vi "Sub Super Duper_7_24_12a_PD.vi"(0 "VISA resource name":refnum<visa-resource-name>="GPIB0::17::INSTR", 1 "Sample Properties:":T5 {"Date Created" format="%<%Y/%m/%d>T"}, 2 "TRF Cluster":T6={"Step 4"=-38.0, "# of Loops"=1.0, "Transfer 2"=FALSE, "Start 4"=-2.0, "Total Points 2"=2, "Start 3"=40.0, "Stop 2"=-40.0, "Step 3"=-1.0, "Loop Step"=0.0, "Integration Time 3"=0, "Loop Wait"=0.0, "First Step"=0.0} {"Loop Wait" format="%<%H:%M:%S>t"; "Integration Time 3" scale=0.0..2.0; "Step 3" format="%.2f"; "Stop 2" format="%.2f"; "Start 3" format="%.2f"; "Start 4" format="%.2f"; "Step 4" format="%.2f"}, 3 "TSP Cluster":T7={"Transport"=FALSE, "Start 2"=0.0, "Stop 3"=-60.0, "Step 2"=-1.0, "Start"=0.0, "Step"=-10.0, "Total Points"=7, "Integration Time"=0} {"Integration Time" scale=0.0..2.0; "Step" format="%.2f"; "Start" format="%.2f"; "Step 2" format="%.2f"; "Stop 3" format="%.2f"; "Start 2" format="%.2f"}, 4 "Compliance Cluster":T2={"Var1 sweep settings"={"sweep spacing (linear: 0)"=0, "sweep mode"=FALSE, "compliance (V)"=100.0, "compliance (A)"=0.001}, "Var1 sweep settings 2"={"sweep spacing (linear: 0)"=0, "sweep mode"=FALSE, "compliance (V)"=100.0, "compliance (A)"=0.001}, "Var2 step settings 2"={"compliance (A)"=0.001, "compliance (V)"=100.0}, "Var2 step settings"={"compliance (A)"=0.001, "compliance (V)"=100.0}} {"Var2 step settings"."compliance (V)" format="%.2f"; "Var2 step settings"."compliance (A)" format="%^.2e"; "Var2 step settings 2"."compliance (V)" format="%.2f"; "Var2 step settings 2"."compliance (A)" format="%^.2e"; "Var1 sweep settings 2"."compliance (A)" format="%^.2e"; "Var1 sweep settings 2"."compliance (V)" format="%.2f"; "Var1 sweep settings 2"."sweep spacing (linear: 0)" items=["linear", "log 10", "log 25", "log 50"]; "Var1 sweep settings"."compliance (A)" format="%^.2e"; "Var1 sweep settings"."compliance (V)" format="%.2f"; "Var1 sweep settings"."sweep spacing (linear: 0)" items=["linear", "log 10", "log 25", "log 50"]}, 5 "error in":errorcluster, 6 "Saved Folder:":path=path "C:/1DATA/2011", 7 "Wait Cluster":T1 {"Wait Time (s)" format="%.1g"; "Wait Countdown" format="%<%H:%M:%S%1u>t"}, 9 "Stop \nCountdown":bool, 11 "Loop Count":dbl) -> (8 "Status Indicator":bool, 14 "VISA resource name out":refnum<visa-resource-name>, 15 "TRF Path":path, 16 "TSP Path":path, 17 "Graph Cluster":T3, 18 "Char Cluster":T4, 19 "error out":errorcluster)   [LabVIEW 2011]
uses:
  <vilib>/Platform/TimedLoop/XDataNode/wakeup.ctl
  <vilib>/Platform/TimedLoop/XDataNode/XDNodeRunTimeDep.lvlib
  <vilib>/Platform/TimedLoop/XDataNode/nitl_modes.ctl
  <vilib>/Platform/TimedLoop/XDataNode/timing_clust.ctl
  <vilib>/Platform/TimedLoop/XDataNode/XDataNode.xnode
panel:
  in  "Transport Temp":cluster{"trace":dbl[], "trace":dbl[]}(graph)
  in  "Graph":cluster{dbl[], "trace":dbl[]}[](graph) caption="Transfer"
  # "Vg Sweep"
  # "Vd Step"
  # "Loops and Integration Time"
  # "Device Characteristics"
  # "Sample Properties:"
  # "%"
  # "nm"
  # "Device Properties:"
  # "um"
  # "um"
  # "Vg Step"
  # "Vd Step"
  # "Integration Time"
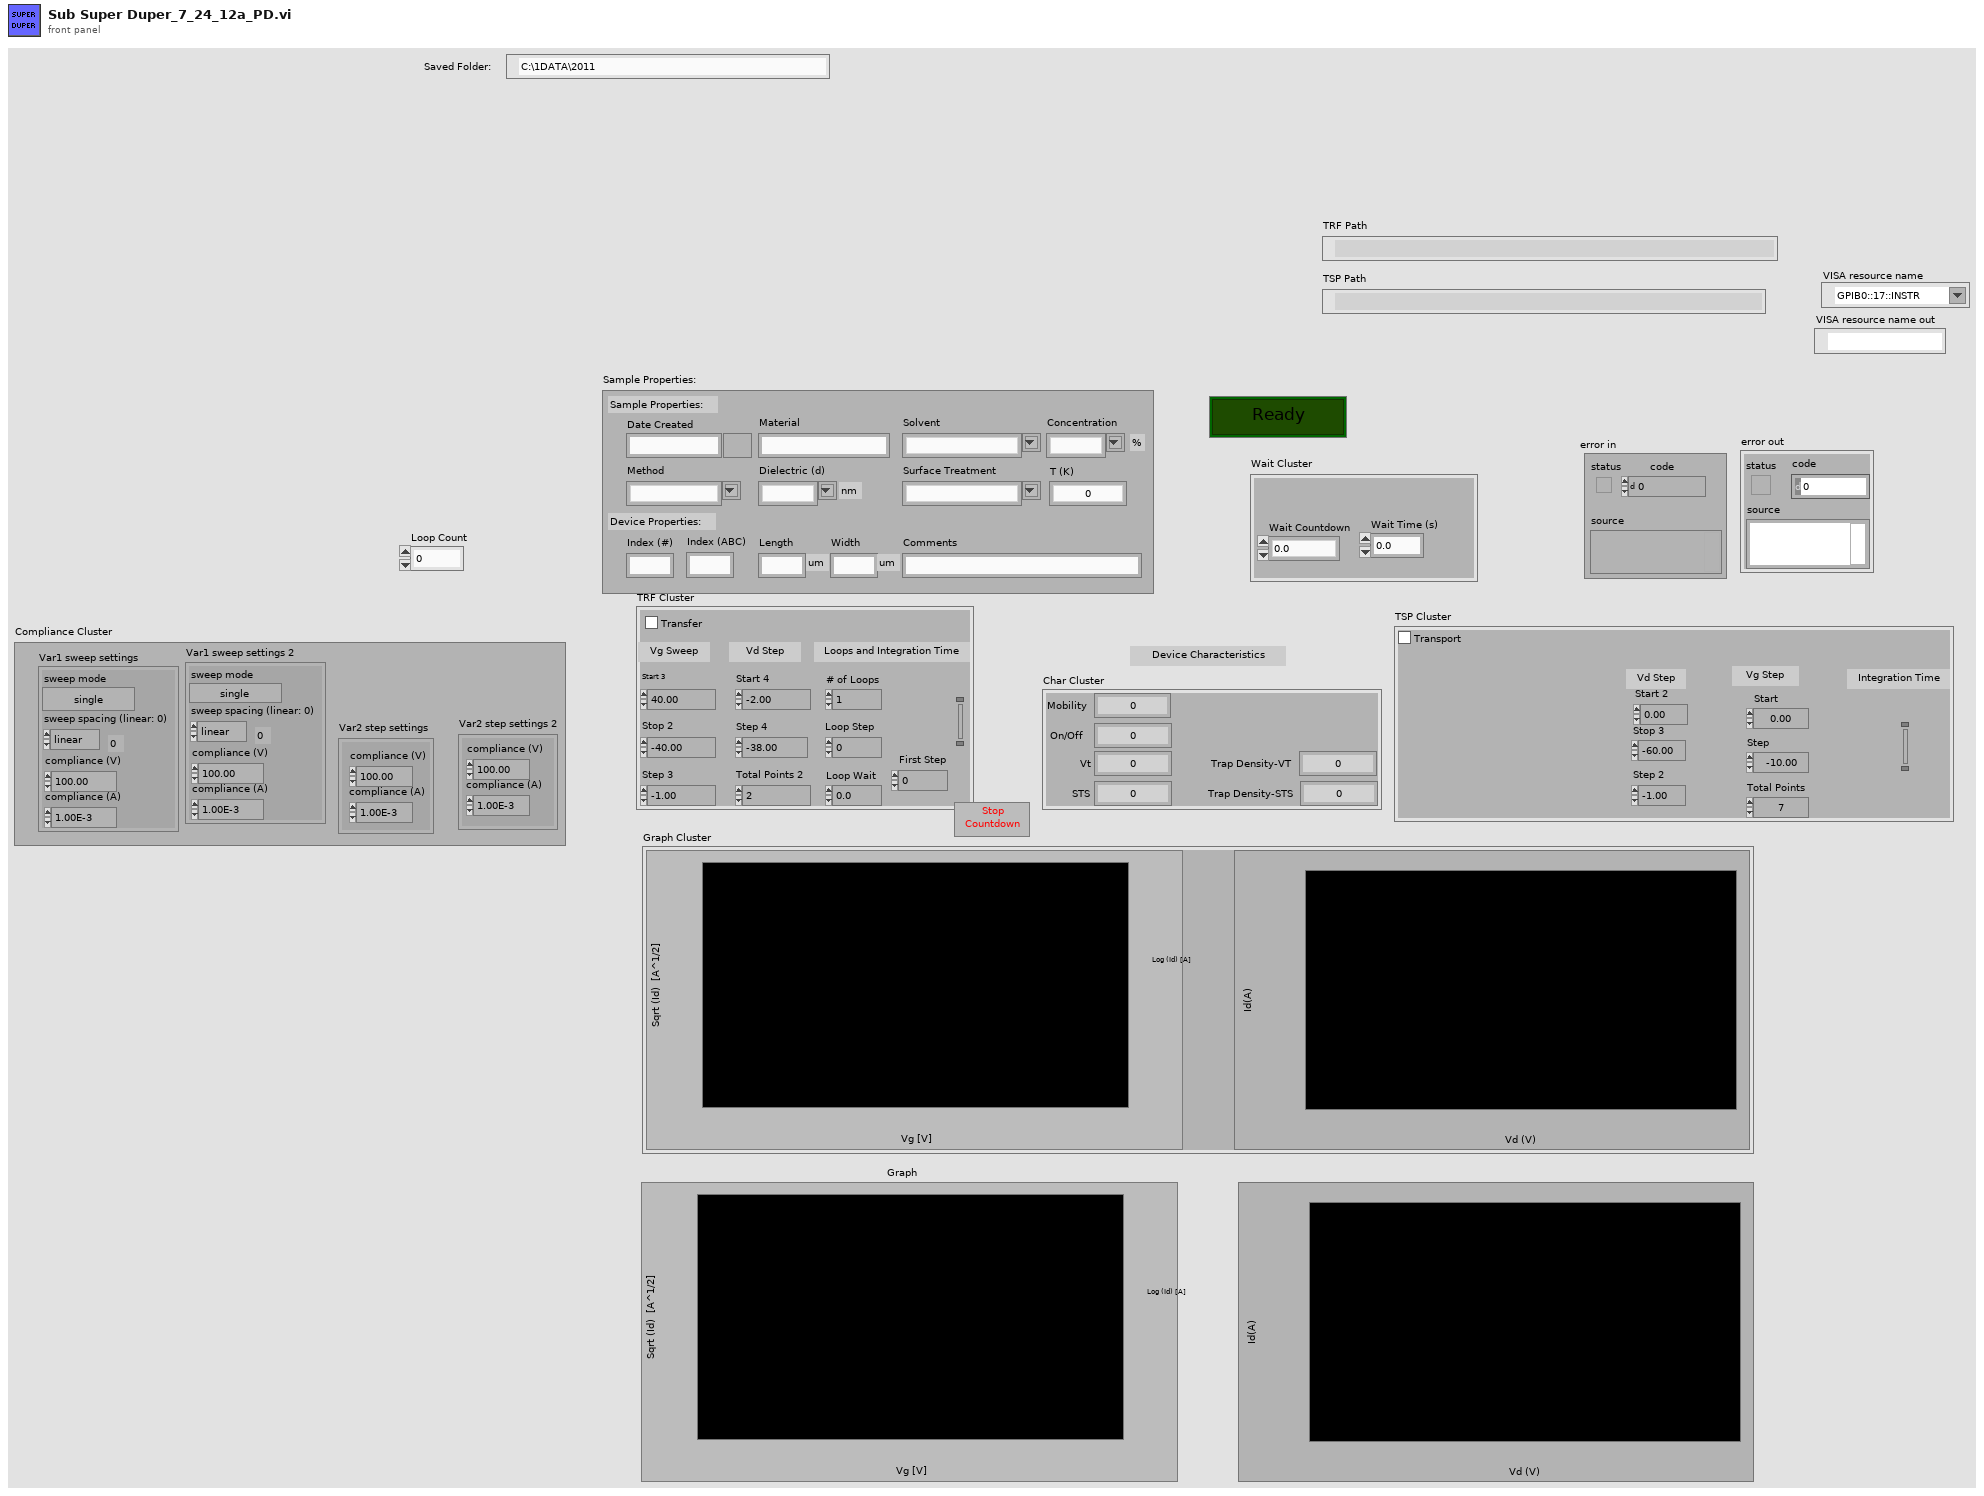
[diagram p1: front panel]
types:
  T1 = cluster{"Wait Countdown":dbl, "Wait Time (s)":dbl}
  T2 = cluster{"Var1 sweep settings":cluster{"sweep spacing (linear: 0)":u16, "sweep mode":bool, "compliance (V)":dbl, "compliance (A)":dbl}, "Var1 sweep settings 2":cluster{"sweep spacing (linear: 0)":u16, "sweep mode":bool, "compliance (V)":dbl, "compliance (A)":dbl}, "Var2 step settings 2":cluster{"compliance (A)":dbl, "compliance (V)":dbl}, "Var2 step settings":cluster{"compliance (A)":dbl, "compliance (V)":dbl}}
  T3 = cluster{"Transfer":cluster{dbl[], "trace":dbl[]}[], "Transport":cluster{"trace":dbl[], "trace":dbl[]}}
  T4 = cluster{"Mobility":dbl, "On/Off ":dbl, "Vt":dbl, "STS":dbl, "Trap Density-STS":dbl, "Trap Density-VT":dbl}
  T5 = cluster{"Date Created":timestamp, "Material":string, "Solvent":string, "Concentration":string, "Method":string, "Dielectric (d)":string, "Index (#)":string, "Index (ABC)":string, "Length":string, "Width":string, "Surface Treatment":string, "Comments":string, "T (K)":dbl}
  T6 = cluster{"Step 4":dbl, "# of Loops":dbl, "Transfer 2":bool, "Start 4":dbl, "Total Points 2":u16, "Start 3":dbl, "Stop 2":dbl, "Step 3":dbl, "Loop Step":dbl, "Integration Time 3":u32, "Loop Wait":dbl, "First Step":dbl}
  T7 = cluster{"Transport":bool, "Start 2":dbl, "Stop 3":dbl, "Step 2":dbl, "Start":dbl, "Step":dbl, "Total Points":u16, "Integration Time":u32}
  T8 = typedef "XDNodeRunTimeDep.lvlib/timing_clust.ctl" = cluster{"Expected End [f-1]":u64, "Actual End [f-1]":u64, "Finished Late? [f-1]":bool, "Expected End [i-1]":u64, "Actual End [i-1]":u64, "Finished Late? [i-1]":bool, "Expected Start [i]":u64, "Actual Start [i]":u64, "Expected Start [f]":u64, "Actual Start [f]":u64, "Source Name":string, "Structure Name":string, "Period":i64, "Deadline":i64, "Offset":i64, "Start":i64, "Priority":i32, "Timeout":i32, "Mode":T9, "Wakeup Reason":T10, "Error":errorcluster, "Source Type":string, "Secondary Source Type":string, "Global End Time":u64, "Global Start Time":u64, "Frame Duration":u64, "Iteration Duration":u64, "Assigned CPU":i32, "I/O Scan Engine Mode":u32}
  T9 = typedef "XDNodeRunTimeDep.lvlib/nitl_modes.ctl" = enum32{"No Change", "Process missed periods, maintain original phase", "Discard missed periods, maintain original phase", "Process missed periods, ignore original phase", "Discard missed periods, ignore original phase"}
  T10 = typedef "XDNodeRunTimeDep.lvlib/wakeup.ctl" = enum32{"Normal", "Aborted", "Asynchronous wakeup", "Timing source error", "Timed loop error", "Timeout"}
  T11 = cluster{"sweep spacing (linear: 0)":u16, "sweep mode":bool, "compliance (V)":dbl, "compliance (A)":dbl}
  T12 = cluster{"compliance (A)":dbl, "compliance (V)":dbl}
  T13 = cluster{"Start 3":dbl, "Stop 2":dbl, "Step 3":dbl, "sweep spacing (linear: 0)":u16, "sweep mode":bool, "compliance (V)":dbl, "compliance (A)":dbl}
  T14 = cluster{"compliance (A)":dbl, "compliance (V)":dbl, "Start 4":dbl, "Total Points 2":u16, dbl}
  T15 = cluster{"Mobility":dbl, "On/Off Current":dbl, "Vt":dbl, "STS":dbl, "Trap Density-VT":dbl, "Trap Density-STS":dbl}
  T16 = cluster{"Start 2":dbl, "Stop 3":dbl, "Step 2":dbl, "sweep spacing (linear: 0)":u16, "sweep mode":bool, "compliance (V)":dbl, "compliance (A)":dbl}
  T17 = cluster{"compliance (A)":dbl, "compliance (V)":dbl, "Start":dbl, "Total Points":u16, "Step":dbl}
  T18 = cluster{"Graph":cluster{dbl[], "trace":dbl[]}[], "Transport Temp":cluster{"trace":dbl[], "trace":dbl[]}}
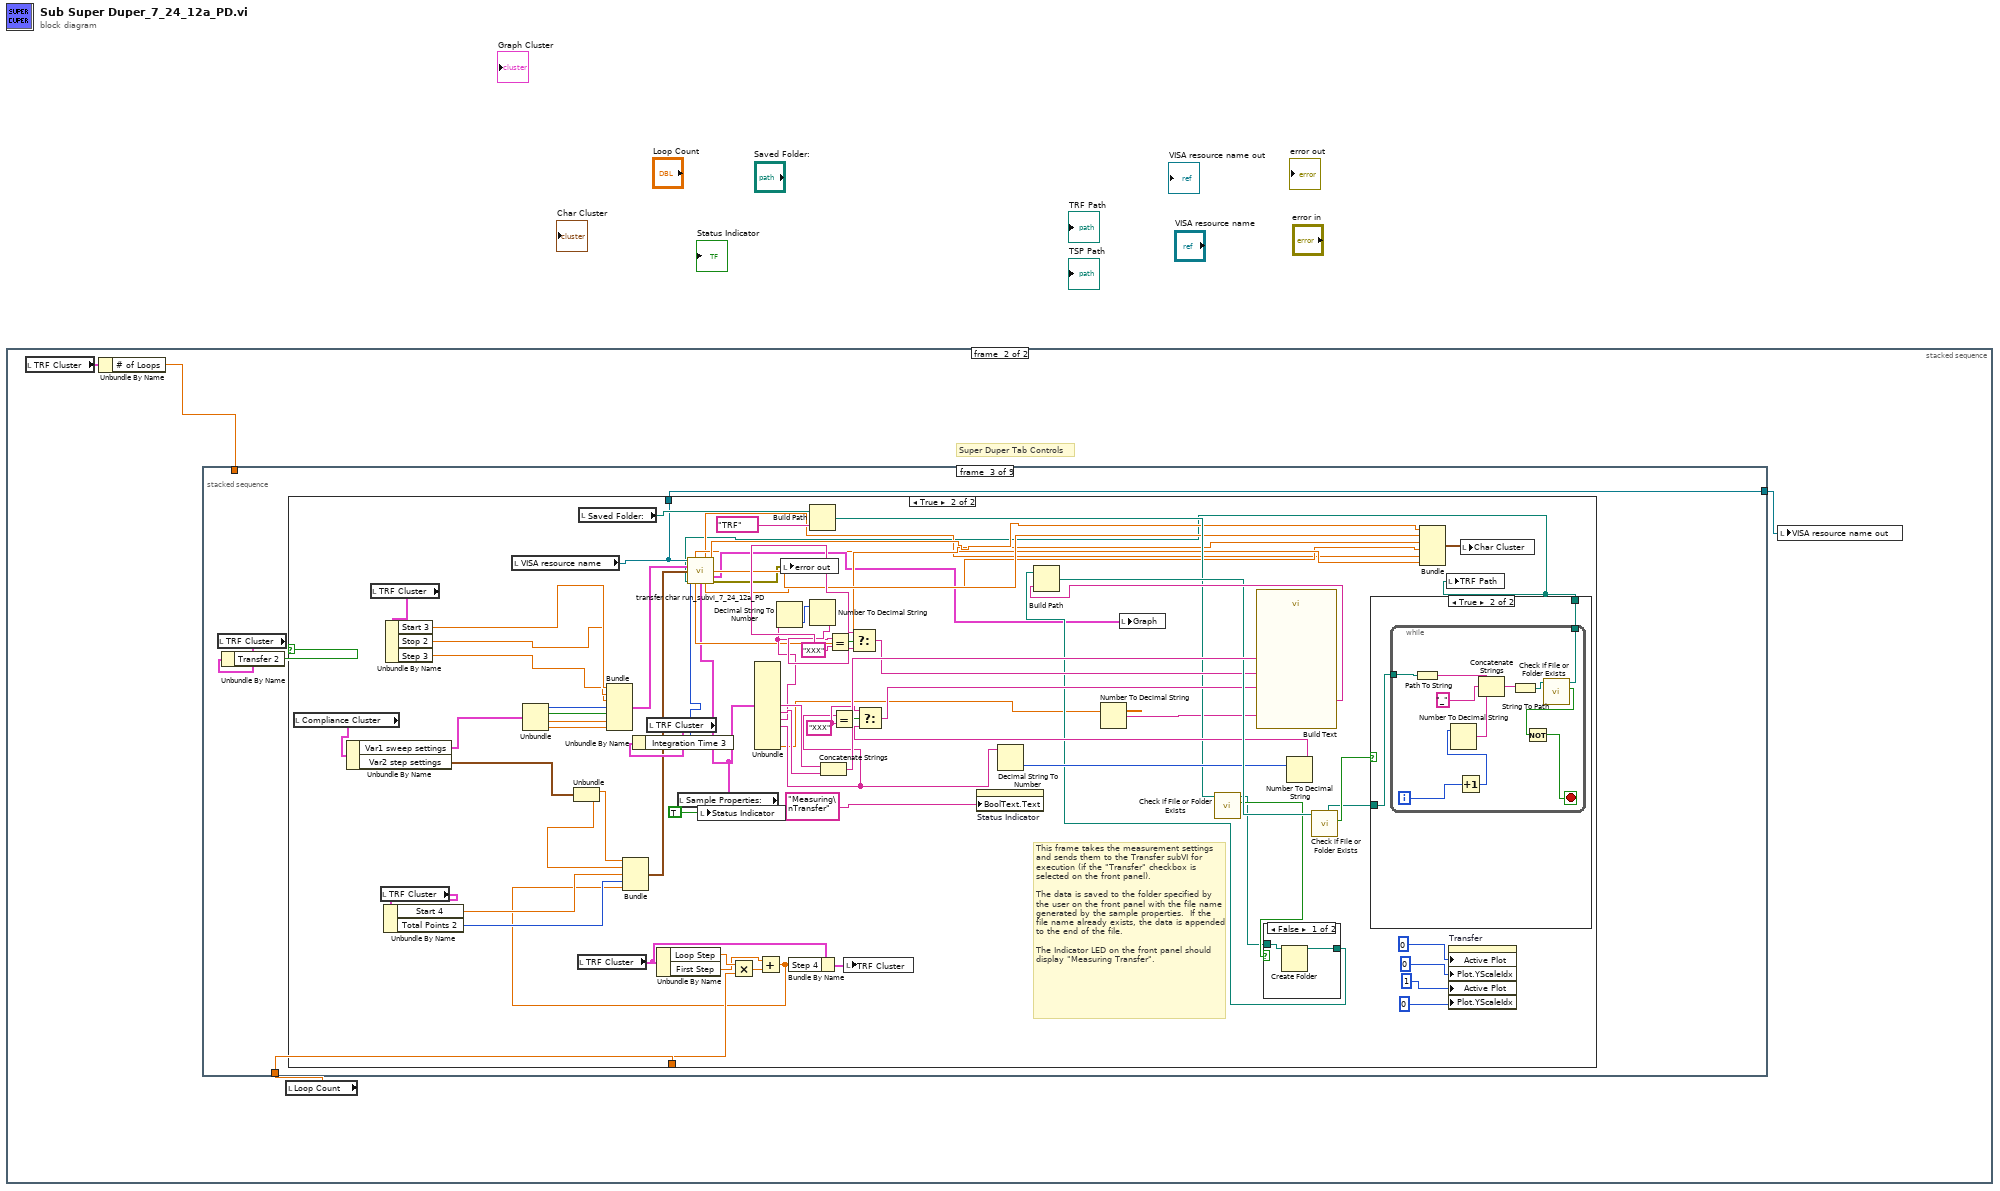
[diagram p0: block diagram]
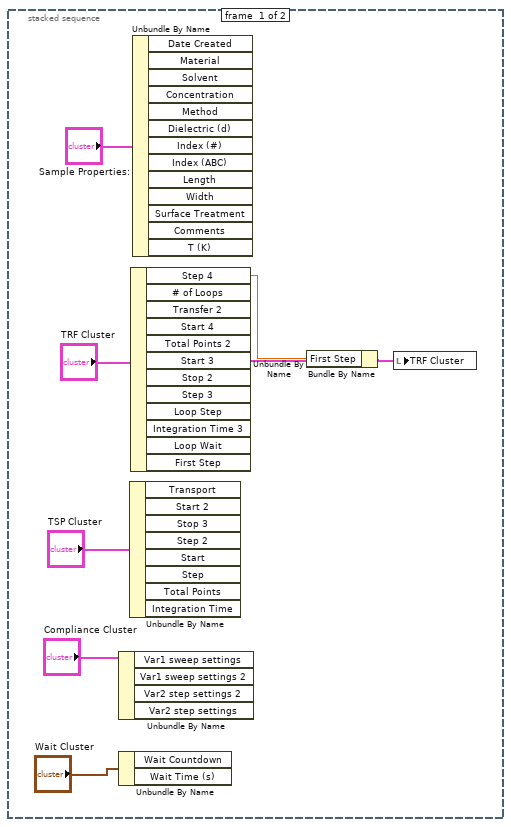
[diagram p2: hidden frame]
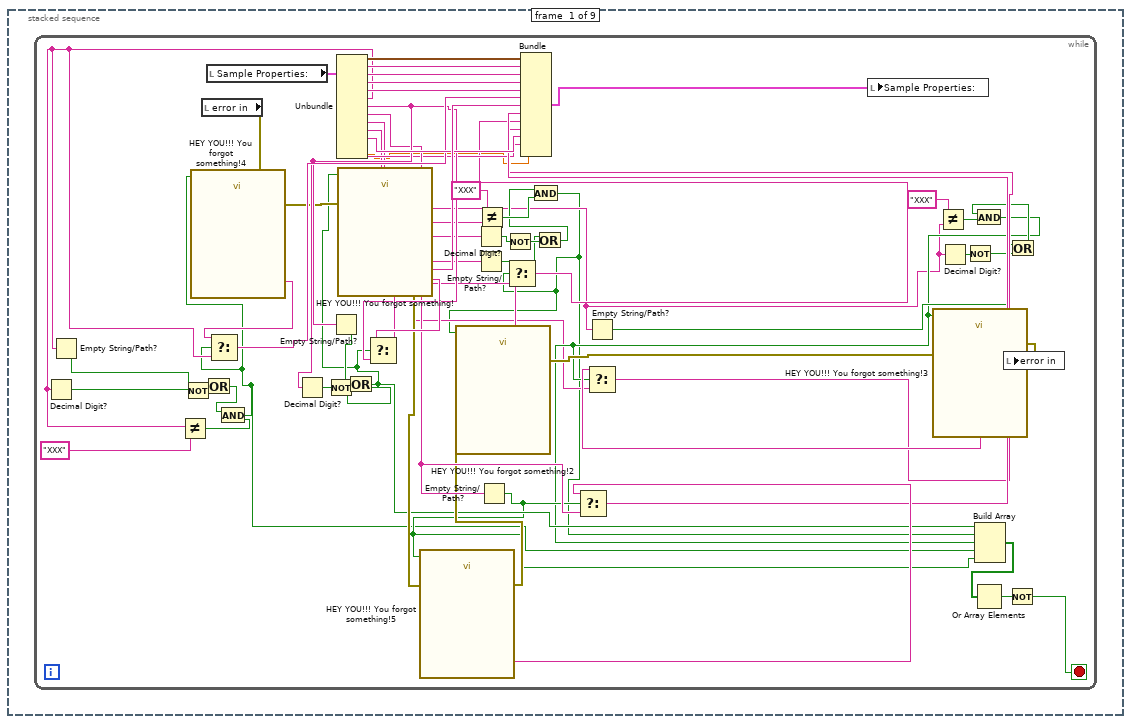
[diagram p3: hidden frame]
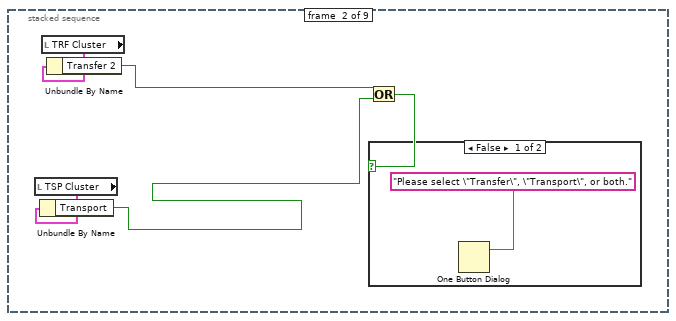
[diagram p4: hidden frame]
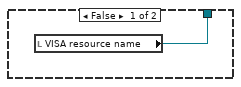
[diagram p6: hidden frame]
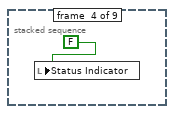
[diagram p9: hidden frame]
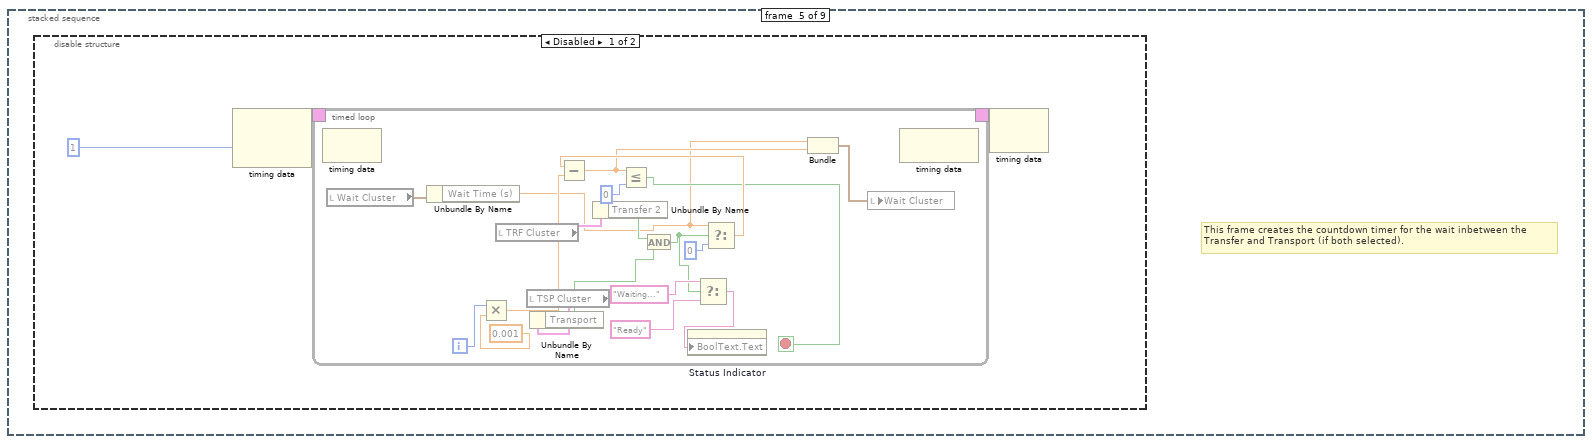
[diagram p10: hidden frame]
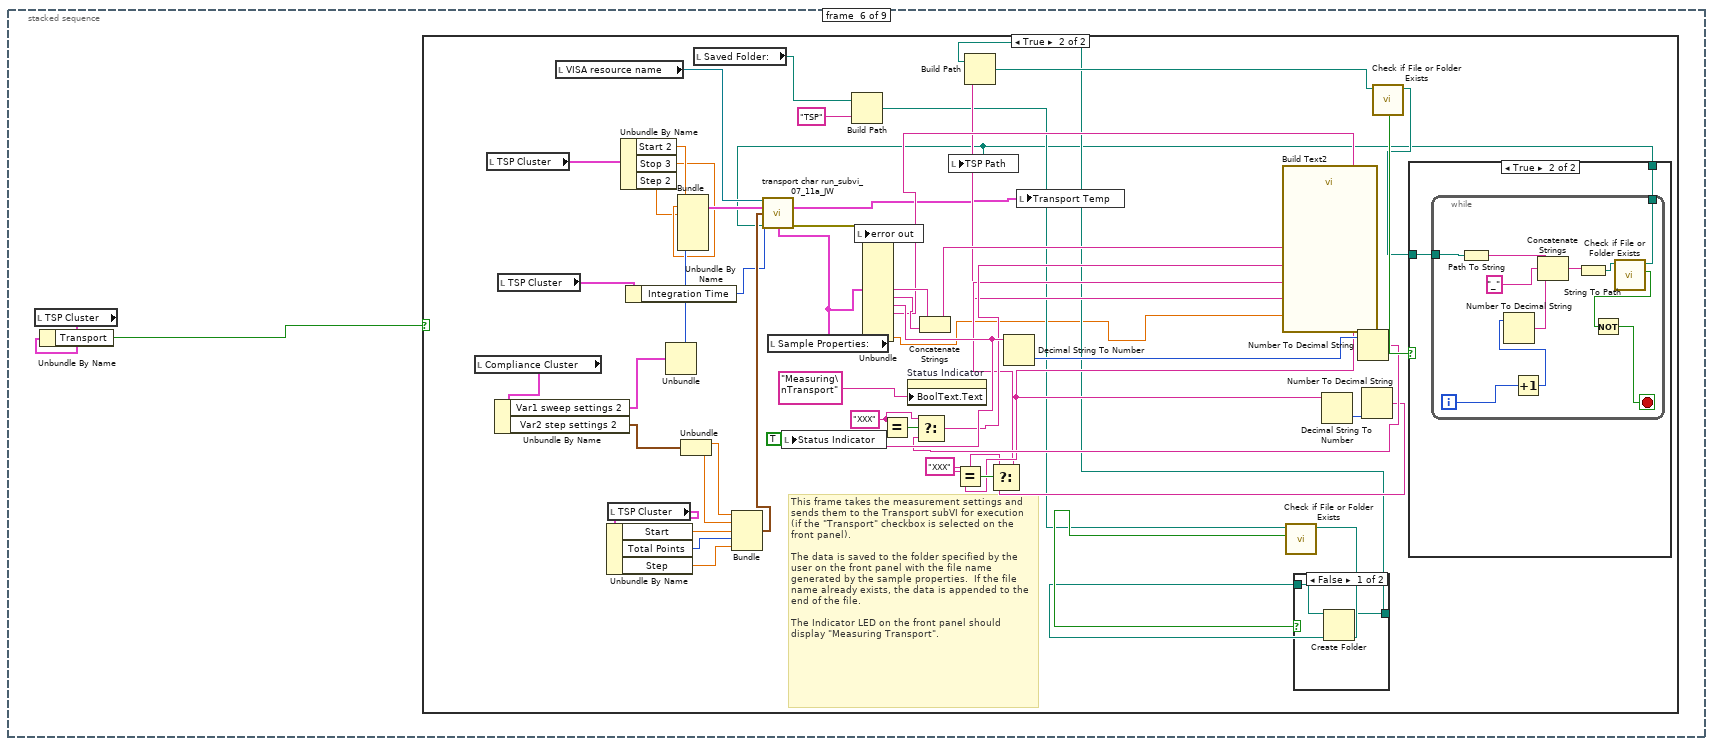
[diagram p12: hidden frame]
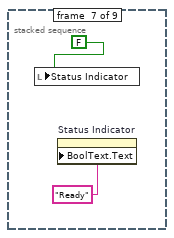
[diagram p16: hidden frame]
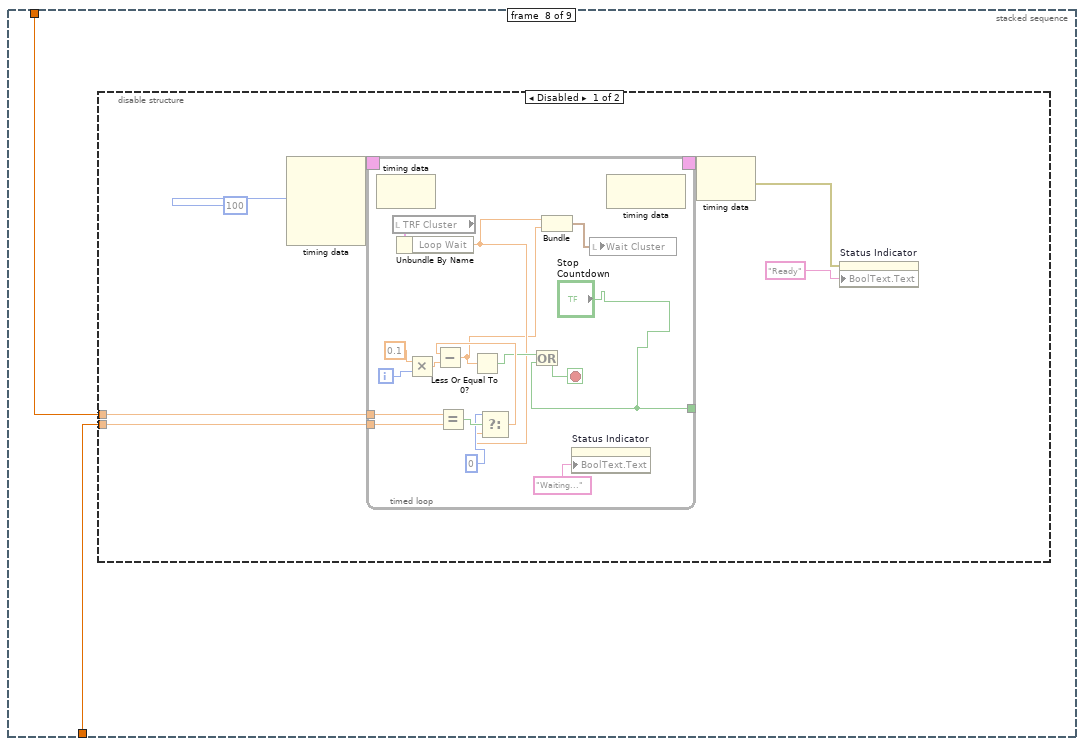
[diagram p17: hidden frame]
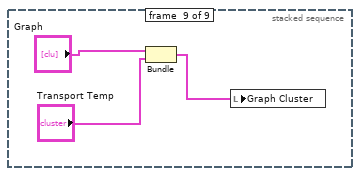
[diagram p19: hidden frame]
diagram:
  n1 = stacked-sequence {
    frame #0 {
      n2 = Unbundle By Name("Compliance Cluster") -> ()  [unwired: 4 out]
      n3 = Unbundle By Name("Wait Cluster") -> ()  [unwired: 2 out]
      n4 = Unbundle By Name("TSP Cluster") -> ()  [unwired: 8 out]
      n5 = Unbundle By Name("TRF Cluster") -> ("Step 4"=w7:dbl)  [unwired: 11 out]
      n6 = Unbundle By Name("Sample Properties:") -> ()  [unwired: 13 out]
      n7 = Bundle By Name(cluster="TRF Cluster", "First Step"=w7) -> (w5:T6)
      n8 = local write "TRF Cluster"(w5) -> ()
    }
    frame #1 {
      # "Super Duper Tab Controls"
      n9 = local read "TRF Cluster"() -> (w11:T6)
      n10 = Unbundle By Name(w11) -> ("# of Loops"=w10:dbl)
      n11 = local read "Loop Count"() -> (w8:dbl)
      n12 = stacked-sequence {
        tunnel: w8 -> [_ _ w81 _ _ _ _ w277 _]
        tunnel: w10 -> [_ _ _ _ _ _ _ w276 _]
        tunnel: [_ _ w78 _ _ _ _ _ _] -> w9
        frame #0 {
          n13 = while {
            stop <- w37 stop-if-true
            n14 = local read "error in"() -> (w43:errorcluster)
            n15 = local read "Sample Properties:"() -> (w66:T5)
            n16 = Unbundle(w66) -> ("Date Created"=w67:timestamp, "Material"=w68:string, "Solvent"=w69:string, "Concentration"=w70:string, "Method"=w71:string, "Dielectric (d)"=w26:string, "Index (#)"=w56:string, "Index (ABC)"=w53:string, "Length"=w21:string, "Width"=w14:string, "Surface Treatment"=w59:string, "Comments"=w51:string, "T (K)"=w12:dbl)
            n17 = Decimal Digit?(1:w26) -> (0:w34:bool)
            n18 = Empty String/Path?(string/path=w26) -> (empty?=w28:bool)
            n19 = Not Equal?(x=w26, y="XXX") -> (x != y?=w25:bool)
            n20 = Not(x=w34) -> (.not. x?=w31:bool)
            n21 = Or(x=w28, y=w31) -> (x .or. y?=w24:bool)
            n22 = And(x=w24, y=w25) -> (x .and. y?=w23:bool)
            n23 = call "HEY YOU!!! You forgot something!4"("Enable"=w23, "error in (no error)"=w43) -> ("Dielectric (d)"=w58:string, "error out"=w42:errorcluster)  [unwired: 15 in, 1 out]
            n24 = Select(t=w58, s=w23, f=w26) -> (s? t:f=w57:string)
            n25 = Decimal Digit?(1:w56) -> (0:w47:bool)
            n26 = Not(x=w47) -> (.not. x?=w46:bool)
            n27 = Empty String/Path?(string/path=w56) -> (empty?=w55:bool)
            n28 = Or(x=w55, y=w46) -> (x .or. y?=w41:bool)
            n29 = call "HEY YOU!!! You forgot something!"("Enable"=w41, "error in (no error)"=w42) -> ("Index (#)"=w65:string, "error out"=w45:errorcluster)  [unwired: 15 in, 1 out]
            n30 = Select(t=w65, s=w41, f=w56) -> (s? t:f=w62:string)
            n31 = Decimal Digit?(1:w21) -> (0:w36:bool)
            n32 = Empty String/Path?(string/path=w21) -> (empty?=w30:bool)
            n33 = Not Equal?(x="XXX", y=w21) -> (x != y?=w20:bool)
            n34 = Empty String/Path?(string/path=w53) -> (empty?=w40:bool)
            n35 = call "HEY YOU!!! You forgot something!5"("Enable"=w40, "error in (no error)"=w45) -> ("Index (ABC)"=w54:string, "error out"=w44:errorcluster)  [unwired: 15 in, 1 out]
            n36 = Not(x=w36) -> (.not. x?=w33:bool)
            n37 = Or(x=w30, y=w33) -> (x .or. y?=w19:bool)
            n38 = And(x=w19, y=w20) -> (x .and. y?=w13:bool)
            n39 = call "HEY YOU!!! You forgot something!2"("Enable"=w13, "error in (no error)"=w44) -> ("Length"=w64:string, "error out"=w61:errorcluster)  [unwired: 15 in, 1 out]
            n40 = Select(t=w64, s=w13, f=w21) -> (s? t:f=w50:string)
            n41 = Select(t=w54, s=w40, f=w53) -> (s? t:f=w52:string)
            n42 = Empty String/Path?(string/path=w14) -> (empty?=w29:bool)
            n43 = Not Equal?(x="XXX", y=w14) -> (x != y?=w18:bool)
            n44 = Decimal Digit?(1:w14) -> (0:w35:bool)
            n45 = Not(x=w35) -> (.not. x?=w32:bool)
            n46 = Or(x=w29, y=w32) -> (x .or. y?=w17:bool)
            n47 = And(x=w17, y=w18) -> (x .and. y?=w16:bool)
            n48 = call "HEY YOU!!! You forgot something!3"("Enable"=w16, "error in (no error)"=w61) -> ("Width"=w63:string, "error out"=w60:errorcluster)  [unwired: 15 in, 1 out]
            n49 = Select(t=w63, s=w16, f=w14) -> (s? t:f=w49:string)
            n50 = Bundle("Date Created"=w67, "Material"=w68, "Solvent"=w69, "Concentration"=w70, "Method"=w71, "Dielectric (d)"=w57, "Index (#)"=w62, "Index (ABC)"=w52, "Length"=w50, "Width"=w49, "Surface Treatment"=w59, "Comments"=w51, "T (K)"=w12) -> (w48:T5)  [unwired: 1 in]
            n51 = local write "Sample Properties:"(w48) -> ()
            n52 = Build Array(w41, w13, w16, w23, w40) -> (w39:bool[])
            n53 = Or Array Elements(Boolean array=w39) -> (logical OR=w38:bool)
            n54 = local write "error in"(w60) -> ()
            n55 = Not(x=w38) -> (.not. x?=w37:bool)
          }
        }
        frame #1 {
          n56 = local read "TSP Cluster"() -> (w73:T7)
          n57 = Unbundle By Name(w73) -> ("Transport"=w72:bool)
          n58 = local read "TRF Cluster"() -> (w75:T6)
          n59 = Unbundle By Name(w75) -> ("Transfer 2"=w74:bool)
          n60 = Or(x=w74, y=w72) -> (x .or. y?=w76:bool)
          n61 = case shown="False" w76 {
            frame False {
              n62 = One Button Dialog(message="Please select \"Transfer\", \"Transport\", or both.") -> ()  [unwired: 1 in, 1 out]
            }
            frame True {
            }
          }
        }
        frame #2 {
          n63 = local read "TRF Cluster"() -> (w79:T6)
          n64 = Unbundle By Name(w79) -> ("Transfer 2"=w80:bool)
          n65 = case shown="True" w80 {
            tunnel: w81 -> [_ w98]
            tunnel: [w82 w89] -> w78
            frame False {
              n66 = local read "VISA resource name"() -> (w82:refnum<visa-resource-name>)
            }
            frame True {
              w132 = "XXX"
              w136 = "XXX"
              # "This frame takes the measurement settings and sends them to the Transfer subVI for execution (if the \"Transfer\" checkbox is selected on the front panel).\n\nThe data is saved to the folder specified by the user on the front panel with the file name generated by the sample properties.  If the file name already exists, the data is appended to the end of the file.\n\nThe Indicator LED on the front panel should display \"Measuring Transfer\"."
              n67 = local read "Compliance Cluster"() -> (w104:T2)
              n68 = Unbundle By Name(w104) -> ("Var1 sweep settings"=w102:T11, "Var2 step settings"=w103:T12)
              n69 = local read "TRF Cluster"() -> (w115:T6)
              n70 = local read "TRF Cluster"() -> (w118:T6)
              n71 = Unbundle By Name(w118) -> ("Start 4"=w117:dbl, "Total Points 2"=w116:u16)
              n72 = Unbundle By Name(w115) -> ("Start 3"=w114:dbl, "Stop 2"=w113:dbl, "Step 3"=w112:dbl)
              n73 = local read "VISA resource name"() -> (w89:refnum<visa-resource-name>)
              n74 = Unbundle(w102) -> ("sweep spacing (linear: 0)"=w154:u16, "sweep mode"=w153:bool, "compliance (V)"=w152:dbl, "compliance (A)"=w151:dbl)
              n75 = Unbundle(w103) -> ("compliance (A)"=w150:dbl, "compliance (V)"=w149:dbl)
              n76 = local read "TRF Cluster"() -> (w93:T6)
              n77 = local read "Saved Folder:"() -> (w105:path)
              n78 = Bundle("Start 3"=w114, "Stop 2"=w113, "Step 3"=w112, "sweep spacing (linear: 0)"=w154, "sweep mode"=w153, "compliance (V)"=w152, "compliance (A)"=w151) -> (w88:T13)  [unwired: 1 in]
              n79 = local read "TRF Cluster"() -> (w111:T6)
              n80 = Unbundle By Name(w111) -> ("Integration Time 3"=w86:u32)
              n81 = Unbundle By Name(w93) -> ("Loop Step"=w96:dbl, "First Step"=w95:dbl)
              n82 = local read "Sample Properties:"() -> (w84:T5)
              n83 = local write "Status Indicator"(TRUE) -> ()
              n84 = Multiply(x=w96, y=w98) -> (x*y=w99:dbl)
              n85 = Unbundle(w84) -> ("Index (#)"=w145:string, "Index (ABC)"=w144:string, "Length"=w128:string, "Width"=w131:string, "T (K)"=w101:dbl)  [unwired: 8 out]
              n86 = Add(x=w95, y=w99) -> (x+y=w94:dbl)
              n87 = Bundle("compliance (A)"=w150, "compliance (V)"=w149, "Start 4"=w117, "Total Points 2"=w116, w94) -> (w87:T14)  [unwired: 1 in]
              n88 = Decimal String To Number(string=w128) -> (number=w139:i32)  [unwired: 2 in, 1 out]
              n89 = Bundle By Name(cluster=w93, "Step 4"=w94) -> (w97:T6)
              n90 = Build Path(base path=w105, name or relative path="TRF") -> (appended path=w124:path)
              n91 = Number To Decimal String(number=w139) -> (decimal integer string=w135:string)  [unwired: 1 in]
              n92 = Concatenate Strings(w145, w144) -> (w143:string)
              n93 = Equal?(x=w128, y=w136) -> (x = y?=w137:bool)
              n94 = Equal?(x=w131, y=w132) -> (x = y?=w133:bool)
              n95 = local write "TRF Cluster"(w97) -> ()
              n96 = Select(t=w136, s=w137, f=w135) -> (s? t:f=w134:string)
              n97 = property on="Status Indicator" class="Bool (strict)"("BoolText.Text"="Measuring\nTransfer") -> ()  [unwired: 2 in, 2 out]
              n98 = Decimal String To Number(string=w131) -> (number=w138:i32)  [unwired: 2 in, 1 out]
              n99 = Number To Decimal String(number=w101) -> (decimal integer string=w100:string)  [unwired: 1 in]
              n100 = call <vilib>:"Check if File or Folder Exists.vi"("path"=w124) -> ("file or folder exists?"=w126:bool, "dup path"=w125:path)  [unwired: 8 in, 1 out]
              n101 = case shown="False" w126 {
                tunnel: w125 -> [w156 w157]
                tunnel: [w155 w157] -> w123
                frame False {
                  n102 = Create Folder(path (use dialog)=w156) -> (created path=w155:path)  [unwired: 2 in, 2 out]
                }
                frame True {
                }
              }
              n103 = Number To Decimal String(number=w138) -> (decimal integer string=w130:string)  [unwired: 1 in]
              n104 = Select(t=w132, s=w133, f=w130) -> (s? t:f=w129:string)
              n105 = call "Build Text"("T"=w100, "Index"=w143, "Length"=w134, "Width"=w129) -> ("Result"=w148:string)  [unwired: 10 in, 1 out]
              n106 = Build Path(base path=w123, name or relative path=w148) -> (appended path=w141:path)
              n107 = call <vilib>:"Check if File or Folder Exists.vi"("path"=w141) -> ("file or folder exists?"=w142:bool, "dup path"=w140:path)  [unwired: 8 in, 1 out]
              n108 = case shown="True" w142 {
                tunnel: w140 -> [w158 w160]
                tunnel: [w158 w159] -> w85
                frame False {
                }
                frame True {
                  n109 = while {
                    tunnel: w160 -> [w162]
                    tunnel: [w161] -> w159
                    i -> [w164]
                    stop <- w165 stop-if-true
                    n110 = Path To String(path=w162) -> (string=w171:string)
                    n111 = Increment(x=w164) -> (x+1=w163:i32)
                    n112 = Number To Decimal String(number=w163) -> (decimal integer string=w169:string)  [unwired: 1 in]
                    n113 = Concatenate Strings(w171, "_", w169) -> (w168:string)
                    n114 = String To Path(string=w168) -> (path=w167:path)
                    n115 = call <vilib>:"Check if File or Folder Exists.vi"("path"=w167) -> ("file or folder exists?"=w166:bool, "dup path"=w161:path)  [unwired: 8 in, 1 out]
                    n116 = Not(x=w166) -> (.not. x?=w165:bool)
                  }
                }
              }
              n117 = call "transfer char run_subvi_7_24_12a_PD.vi"("VISA session"=w89, "Var1 sweep settings"=w88, "Var2 step settings"=w87, "integration time"=w86, "Input Path"=w85, "Sample Properties:"=w84) -> ("Trap Density-STS"=w92:dbl, "Trap Density-VT"=w90:dbl, "Mobility"=w109:dbl, "On/Off Current"=w108:dbl, "XY Graph"=w106:cluster{dbl[], "trace":dbl[]}[], "Vt"=w107:dbl, "STS"=w91:dbl, "error?"=w83:errorcluster)  [unwired: 1 in, 1 out]
              n118 = local write "error out"(w83) -> ()
              n119 = local write "Graph"(w106) -> ()
              n120 = Bundle("Mobility"=w109, "On/Off Current"=w108, "Vt"=w107, "STS"=w91, "Trap Density-VT"=w90, "Trap Density-STS"=w92) -> (w110:T15)  [unwired: 1 in]
              n121 = local write "TRF Path"(w85) -> ()
              n122 = property on="Transfer" class="XYGraph (strict)"("Active Plot"=0, "Plot.YScaleIdx"=0, "Active Plot"=1, "Plot.YScaleIdx"=0) -> ()  [unwired: 2 in, 2 out]
              n123 = local write "Char Cluster"(w110) -> ()
            }
          }
        }
        frame #3 {
          n124 = local write "Status Indicator"(FALSE) -> ()
        }
        frame #4 {
          # "This frame creates the countdown timer for the wait inbetween the\nTransfer and Transport (if both selected)."
          n125 = disable-structure shown="Disabled" {
            frame Disabled {
              n126 = node-c288(1) -> (w175:T8)  [unwired: 1 in]
              n127 = timed-loop {
                timing: w175 -> [_]
                timing-out: [_] -> w174
                i -> [w186]
                stop <- w187 stop-if-true
                n128 = node-c288() -> ()  [unwired: 1 in, 1 out]
                n129 = local read "Wait Cluster"() -> (w179:T1)
                n130 = Unbundle By Name(w179) -> ("Wait Time (s)"=w177:dbl)
                n131 = Multiply(x=w186, y=0.001) -> (x*y=w184:dbl)
                n132 = local read "TRF Cluster"() -> (w180:T6)
                n133 = local read "TSP Cluster"() -> (w181:T7)
                n134 = Unbundle By Name(w181) -> ("Transport"=w182:bool)
                n135 = Unbundle By Name(w180) -> ("Transfer 2"=w183:bool)
                n136 = And(x=w183, y=w182) -> (x .and. y?=w191:bool)
                n137 = Select(t="Waiting...", s=w191, f="Ready") -> (s? t:f=w193:string)
                n138 = property on="Status Indicator" class="Bool (strict)"("BoolText.Text"=w193) -> ()  [unwired: 2 in, 2 out]
                n139 = Select(t=w177, s=w191, f=0) -> (s? t:f=w189:dbl)
                n140 = Subtract(x=w189, y=w184) -> (x-y=w178:dbl)
                n141 = Less Or Equal?(x=w178, y=0) -> (x <= y?=w187:bool)
                n142 = Bundle("Wait Time (s)"=w177, w178) -> (w176:cluster{"Wait Time (s)":dbl, dbl})  [unwired: 1 in]
                n143 = local write "Wait Cluster"(w176) -> ()
                n144 = node-c288() -> ()  [unwired: 1 in, 1 out]
              }
              n145 = node-c288(w174) -> ()  [unwired: 1 out]
            }
            frame Enabled {
            }
          }
        }
        frame #5 {
          n146 = local read "TSP Cluster"() -> (w202:T7)
          n147 = Unbundle By Name(w202) -> ("Transport"=w201:bool)
          n148 = case shown="True" w201 {
            frame False {
            }
            frame True {
              w229 = "XXX"
              w233 = "XXX"
              # "This frame takes the measurement settings and sends them to the Transport subVI for execution (if the \"Transport\" checkbox is selected on the front panel).\n\nThe data is saved to the folder specified by the user on the front panel with the file name generated by the sample properties.  If the file name already exists, the data is appended to the end of the file.\n\nThe Indicator LED on the front panel should display \"Measuring Transport\"."
              n149 = local read "Compliance Cluster"() -> (w207:T2)
              n150 = local read "TSP Cluster"() -> (w220:T7)
              n151 = Unbundle By Name(w207) -> ("Var1 sweep settings 2"=w206:T11, "Var2 step settings 2"=w205:T12)
              n152 = local read "TSP Cluster"() -> (w213:T7)
              n153 = local read "VISA resource name"() -> (w209:refnum<visa-resource-name>)
              n154 = local read "TSP Cluster"() -> (w211:T7)
              n155 = Unbundle By Name(w211) -> ("Start"=w216:dbl, "Total Points"=w215:u16, "Step"=w214:dbl)
              n156 = Unbundle By Name(w220) -> ("Start 2"=w219:dbl, "Stop 3"=w218:dbl, "Step 2"=w217:dbl)
              n157 = Unbundle By Name(w213) -> ("Integration Time"=w212:u32)
              n158 = Unbundle(w206) -> ("sweep spacing (linear: 0)"=w256:u16, "sweep mode"=w255:bool, "compliance (V)"=w254:dbl, "compliance (A)"=w253:dbl)
              n159 = Bundle("Start 2"=w219, "Stop 3"=w218, "Step 2"=w217, "sweep spacing (linear: 0)"=w256, "sweep mode"=w255, "compliance (V)"=w254, "compliance (A)"=w253) -> (w252:T16)  [unwired: 1 in]
              n160 = Unbundle(w205) -> ("compliance (A)"=w251:dbl, "compliance (V)"=w250:dbl)
              n161 = local read "Saved Folder:"() -> (w208:path)
              n162 = Bundle("compliance (A)"=w251, "compliance (V)"=w250, "Start"=w216, "Total Points"=w215, "Step"=w214) -> (w249:T17)  [unwired: 1 in]
              n163 = local read "Sample Properties:"() -> (w245:T5)
              n164 = local write "Status Indicator"(TRUE) -> ()
              n165 = Build Path(base path=w208, name or relative path="TSP") -> (appended path=w222:path)
              n166 = Unbundle(w245) -> ("Index (#)"=w244:string, "Index (ABC)"=w243:string, "Length"=w234:string, "Width"=w230:string, "T (K)"=w203:dbl)  [unwired: 8 out]
              n167 = Equal?(x=w233, y=w234) -> (x = y?=w235:bool)
              n168 = property on="Status Indicator" class="Bool (strict)"("BoolText.Text"="Measuring\nTransport") -> ()  [unwired: 2 in, 2 out]
              n169 = Concatenate Strings(w244, w243) -> (w242:string)
              n170 = Equal?(x=w229, y=w230) -> (x = y?=w238:bool)
              n171 = Decimal String To Number(string=w234) -> (number=w237:i32)  [unwired: 2 in, 1 out]
              n172 = call <vilib>:"Check if File or Folder Exists.vi"("path"=w222) -> ("file or folder exists?"=w224:bool, "dup path"=w223:path)  [unwired: 8 in, 1 out]
              n173 = case shown="False" w224 {
                tunnel: w223 -> [w258 w259]
                tunnel: [w257 w259] -> w221
                frame False {
                  n174 = Create Folder(path (use dialog)=w258) -> (created path=w257:path)  [unwired: 2 in, 2 out]
                }
                frame True {
                }
              }
              n175 = Decimal String To Number(string=w230) -> (number=w236:i32)  [unwired: 2 in, 1 out]
              n176 = Number To Decimal String(number=w237) -> (decimal integer string=w232:string)  [unwired: 1 in]
              n177 = Select(t=w233, s=w235, f=w232) -> (s? t:f=w231:string)
              n178 = Number To Decimal String(number=w236) -> (decimal integer string=w228:string)  [unwired: 1 in]
              n179 = Select(t=w229, s=w238, f=w228) -> (s? t:f=w227:string)
              n180 = call "Build Text2"("T"=w203, "Index"=w242, "Length"=w231, "Width"=w227) -> ("Result"=w226:string)  [unwired: 10 in, 1 out]
              n181 = Build Path(base path=w221, name or relative path=w226) -> (appended path=w239:path)
              n182 = call <vilib>:"Check if File or Folder Exists.vi"("path"=w239) -> ("file or folder exists?"=w241:bool, "dup path"=w240:path)  [unwired: 8 in, 1 out]
              n183 = case shown="True" w241 {
                tunnel: w240 -> [w260 w262]
                tunnel: [w260 w261] -> w204
                frame False {
                }
                frame True {
                  n184 = while {
                    tunnel: w262 -> [w264]
                    tunnel: [w263] -> w261
                    i -> [w266]
                    stop <- w267 stop-if-true
                    n185 = Path To String(path=w264) -> (string=w273:string)
                    n186 = Increment(x=w266) -> (x+1=w265:i32)
                    n187 = Number To Decimal String(number=w265) -> (decimal integer string=w271:string)  [unwired: 1 in]
                    n188 = Concatenate Strings(w273, "_", w271) -> (w270:string)
                    n189 = String To Path(string=w270) -> (path=w269:path)
                    n190 = call <vilib>:"Check if File or Folder Exists.vi"("path"=w269) -> ("file or folder exists?"=w268:bool, "dup path"=w263:path)  [unwired: 8 in, 1 out]
                    n191 = Not(x=w268) -> (.not. x?=w267:bool)
                  }
                }
              }
              n192 = call "transport char run_subvi_07_11a_JW.vi"("VISA session"=w209, "Var1 sweep settings"=w252, "Var2 step settings"=w249, "integration time"=w212, "Path"=w204, "Sample Properties:"=w245) -> ("graphic display"=w210:cluster{"trace":dbl[], "trace":dbl[]}, "error?"=w248:errorcluster)  [unwired: 8 in]
              n193 = local write "error out"(w248) -> ()
              n194 = local write "TSP Path"(w204) -> ()
              n195 = local write "Transport Temp"(w210) -> ()
            }
          }
        }
        frame #6 {
          n196 = local write "Status Indicator"(FALSE) -> ()
          n197 = property on="Status Indicator" class="Bool (strict)"("BoolText.Text"="Ready") -> ()  [unwired: 2 in, 2 out]
        }
        frame #7 {
          n198 = disable-structure shown="Disabled" {
            disable-tunnel: w277 -> [w279 _]
            disable-tunnel: w276 -> [w278 _]
            frame Disabled {
              n199 = node-c288(100) -> (w284:T8)  [unwired: 3 in]
              n200 = timed-loop {
                timing: w284 -> [_]
                timing-out: [_] -> w283
                tunnel: w279 -> [w295]
                tunnel: w278 -> [w294]
                tunnel: ["Stop \nCountdown"] -> _
                i -> [w300]
                stop <- w290 stop-if-true
                n201 = node-c288() -> ()  [unwired: 1 in, 1 out]
                n202 = local read "TRF Cluster"() -> (w289:T6)
                n203 = Unbundle By Name(w289) -> ("Loop Wait"=w287:dbl)
                n204 = Multiply(x=0.1, y=w300) -> (x*y=w298:dbl)
                n205 = Equal?(x=w294, y=w295) -> (x = y?=w296:bool)
                n206 = Select(t=0, s=w296, f=w287) -> (s? t:f=w292:dbl)
                n207 = Subtract(x=w292, y=w298) -> (x-y=w286:dbl)
                n208 = Less Or Equal To 0?(x=w286) -> (x <= 0?=w291:bool)
                n209 = Or(x=w291, y="Stop \nCountdown") -> (x .or. y?=w290:bool)
                n210 = Bundle("Loop Wait"=w287, w286) -> (w288:cluster{"Loop Wait":dbl, dbl})  [unwired: 1 in]
                n211 = property on="Status Indicator" class="Bool (strict)"("BoolText.Text"="Waiting...") -> ()  [unwired: 2 in, 2 out]
                n212 = local write "Wait Cluster"(w288) -> ()
                n213 = node-c288() -> ()  [unwired: 1 in, 1 out]
              }
              n214 = node-c288(w283) -> (w280:errorcluster)
              n215 = property on="Status Indicator" class="Bool (strict)"(error in=w280, "BoolText.Text"="Ready") -> ()  [unwired: 1 in, 2 out]
            }
            frame Enabled {
            }
          }
        }
        frame #8 {
          n216 = Bundle("Graph"="Graph", "Transport Temp"="Transport Temp") -> (w310:T18)  [unwired: 1 in]
          n217 = local write "Graph Cluster"(w310) -> ()
        }
      }
      n218 = local write "VISA resource name out"(w9) -> ()
    }
  }
